vi "Initialize.vi"(8 "error in":errorcluster) -> (0 "error out":errorcluster, 3 "CoreOOB_Rx out":refnum<class "CIFTemplateCoreOOB_Rx.lvclass">)   [LabVIEW 2021, in "CIFTemplateCoreOOB_Rx.lvclass"]
uses:
  CIFTemplateCoreOOB_Rx.lvclass
  D:/dev/CIF-Core-LabVIEW/src/CIFUtilities/CifOutOfBand/CIFOutOfBand.lvclass
  CIFTemplateCommon/Typedef/Common Plugin Configuration.ctl
  Typedef/Template Payload.ctl
  CIFUtilities/CifOutOfBand/CIFOutOfBand.lvclass/CIFOutOfBand.ctl
  CIFTemplateCoreOOB_Rx.lvclass/CIFTemplateCoreOOB_Rx.ctl
  CIFUtilities/CifOutOfBand/CIFOutOfBand.lvclass
  CIFTemplateCommon/CIFTemplateCommon.lvlib
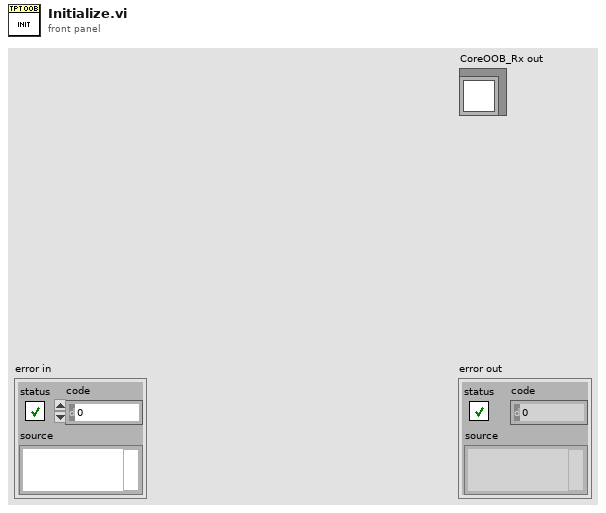
[diagram p1: front panel]
types:
  T1 = typedef "CIFTemplateCoreOOB_Rx.lvclass/Template Payload.ctl" = cluster{"Config Data":variant, "FTE":u64}
  T2 = typedef "CIFTemplateCommon.lvlib/Common Plugin Configuration.ctl" = cluster{"Iteration Interval (s)":dbl, "T0 (ns)":u64, "Priority":i32, "Processor":i32}
  T3 = typedef "CIFTemplateCoreOOB_Rx.lvclass/Command Setting Control.ctl" = cluster{"Enum":T4, "U8":u8, " Payload":bool}
  T4 = typedef "CIFTemplateCoreOOB_Rx.lvclass/OOB Core Commands.ctl" = enum8{"Start", "StartFTE", "Pause", "Stop", "Restart", "RestartFTE", "RefreshStats", "UpdateConfig"}
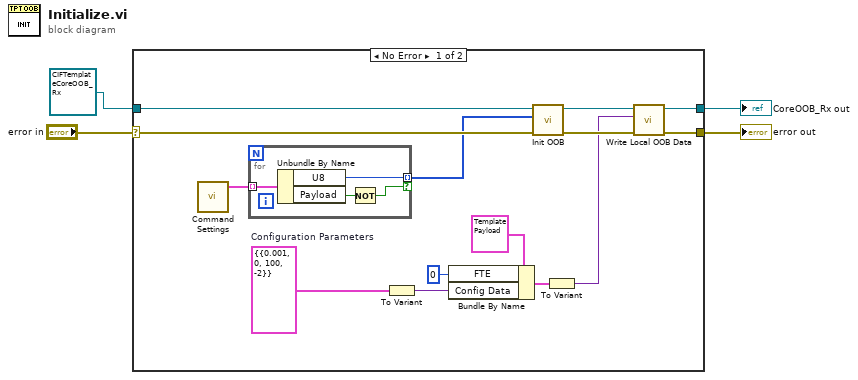
[diagram p0: block diagram]
diagram:
  n1 = case shown="No Error" "error in" {
    selector: "error in" -> [w18 w24]
    tunnel: [w11 w24] -> w3
    tunnel: [w12 w23] -> w2
    tunnel: refnum<class "CIFTemplateCoreOOB_Rx.lvclass"> refnum ("CifLvTemplateOutOfBand in") -> [w17 w23]
    frame No Error {
      w6 = cluster{"Common":T2} {"Common"={"Iteration Interval (s)"=0.001, "T0 (ns)"=0, "Priority"=100, "Processor"=-2}}  # Configuration Parameters
      n2 = call "Command Settings.vi"() -> ("Command Settings"=w16:T3[])  [unwired: 5 in]
      n3 = for {
        tunnel: w16 -> [w22] mode=indexing
        tunnel: [w21] -> w15 mode=indexing if=w19
        n4 = Unbundle By Name(w22) -> ("U8"=w21:u8, "Payload"=w20:bool)
        n5 = Not(x=w20) -> (.not. x?=w19:bool)
      }
      n6 = To Variant(anything=w6) -> (Variant=w5:variant)
      n7 = Bundle By Name(cluster=T1 {"Config Data"=variant, "FTE"=0} ("Template Payload"), "FTE"=u64 0, "Config Data"=w5) -> (w9:T1)
      n8 = call "Init OOB.vi"("error in (no error)"=w18, "Cases to Skip Payload"=w15, "OOB in"=w17) -> ("error out"=w14:errorcluster, "OOB out"=w13:refnum<class "CIFTemplateCoreOOB_Rx.lvclass">)  [unwired: 7 in]
      n9 = To Variant(anything=w9) -> (Variant=w8:variant)
      n10 = call "Write Local OOB Data.vi"("error in"=w14, "Local OOB Data"=w8, "OOB in"=w13) -> ("error out"=w11:errorcluster, "OOB out"=w12:refnum<class "CIFTemplateCoreOOB_Rx.lvclass">)  [unwired: 7 in]
    }
    frame Error {
    }
  }
  "error out" <- w3
  "CoreOOB_Rx out" <- w2
